vi "Filter for Reports.vi"(7 "Action class name (\"\" = Disable)":string, 8 "error in (no error)":errorcluster, 9 "Type filter (Report = Disable)":T1, 10 "Action Number(<0 = Disable)":i32=-1, 11 "Project Builder in":refnum<class "Project Builder.lvclass">) -> (0 "error out":errorcluster, 1 "Match Found?":bool, 2 "Match Count":i32, 3 "Filtered Reports":T2[](array[typedef]) {"Time End" format="%<%x %.3X>T"; "Time Start" format="%<%x %.3X>T"})   [LabVIEW 2020, in "ProjectBuilder.lvlib" / "Project Builder.lvclass"]
uses:
  Project Builder.lvclass
  Data/Report Data/Report Data.lvclass
  Action/Project Action/Project Action.lvclass
  Ctl/Ctl_Build Steps.ctl
  ProjectBuilder.lvlib
  Ctl/Ctl_Action Result.ctl
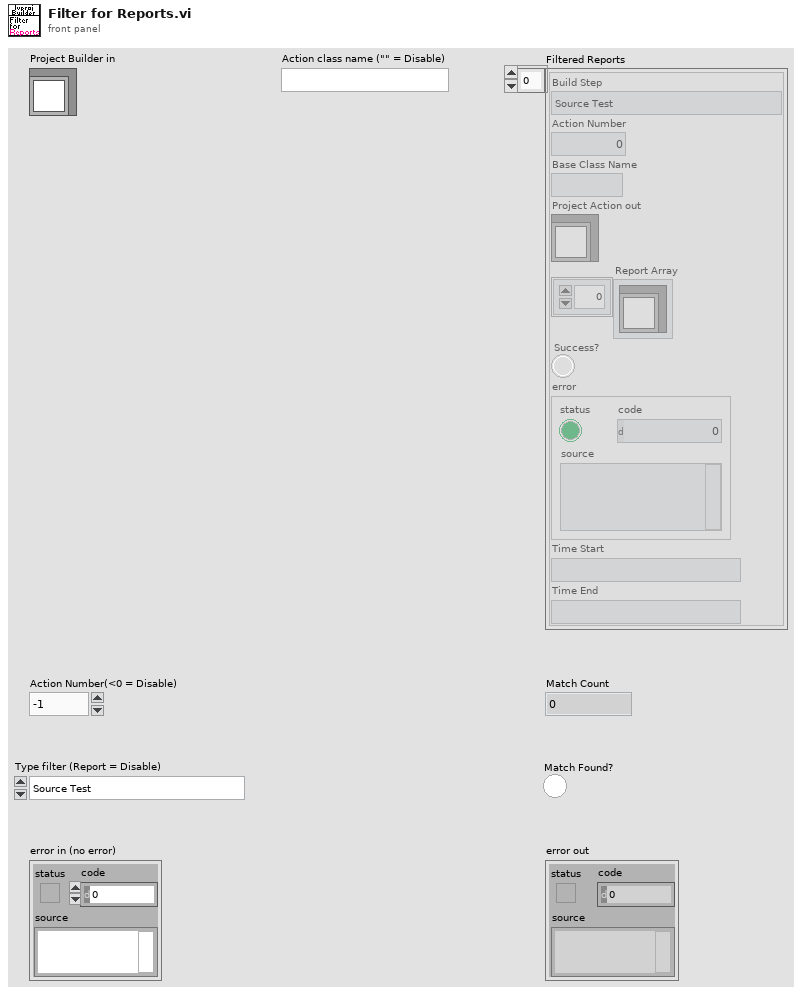
[diagram p1: front panel]
types:
  T1 = typedef "ProjectBuilder.lvlib/Ctl_Build Steps.ctl" = enum16{"Source Test", "Build", "Post-Build Test", "Deploy", "Report"}
  T2 = typedef "ProjectBuilder.lvlib/Ctl_Action Result.ctl" = cluster{"Build Step":T1, "Action Number":i32, "Base Class Name":string, "Project Action out":refnum<class "Project Action.lvclass">, "Report Array":refnum<class "Report Data.lvclass">[], "Success?":bool, "error":errorcluster, "Time Start":timestamp, "Time End":timestamp}
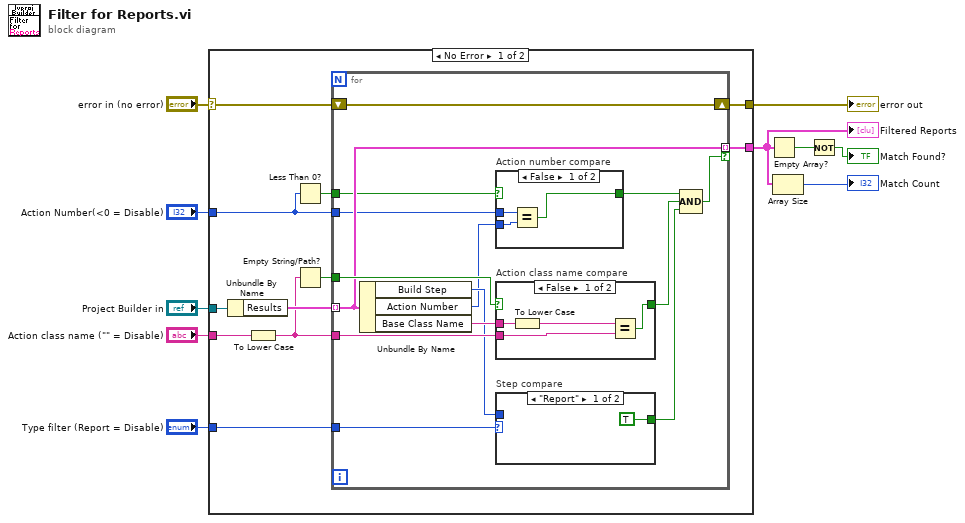
[diagram p0: block diagram]
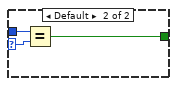
[diagram p3: hidden frame]
diagram:
  n1 = case shown="No Error" "error in (no error)" {
    selector: "error in (no error)" -> [w14 w49]
    tunnel: [w13 w49] -> w9
    tunnel: "Project Builder in" -> [w21 _]
    tunnel: "Action class name (\"\" = Disable)" -> [w19 _]
    tunnel: [w16 _] -> w4
    tunnel: "Type filter (Report = Disable)" -> [w15 _]
    tunnel: "Action Number(<0 = Disable)" -> [w11 _]
    frame No Error {
      n2 = Unbundle By Name(w21) -> ("Results"=w20:T2[])
      n3 = To Lower Case(string=w19) -> (all lower case string=w18:string)
      n4 = Less Than 0?(x=w11) -> (x < 0?=w12:bool)
      n5 = Empty String/Path?(string/path=w18) -> (empty?=w17:bool)
      n6 = for {
        tunnel: w20 -> [w31] mode=indexing
        tunnel: w18 -> [w33]
        tunnel: w17 -> [w34]
        tunnel: [w31] -> w16 mode=indexing if=w30
        tunnel: w15 -> [w29]
        shift-right: [w26] -> w13
        shift-left: w14 -> [w26]
        tunnel: w12 -> [w25]
        tunnel: w11 -> [w23]
        n7 = Unbundle By Name(w31) -> ("Build Step"=w27:T1, "Action Number"=w22:i32, "Base Class Name"=w35:string)
        n8 = case "Action number compare" shown="False" w25 {
          selector: w25 -> [_ w39]
          tunnel: [w36 w39] -> w24
          tunnel: w23 -> [w38 _]
          tunnel: w22 -> [w37 _]
          frame False {
            n9 = Equal?(x=w38, y=w37) -> (x = y?=w36:bool)
          }
          frame True {
          }
        }
        n10 = case "Action class name compare" shown="False" w34 {
          selector: w34 -> [_ w48]
          tunnel: w35 -> [w47 _]
          tunnel: w33 -> [w45 _]
          tunnel: [w44 w48] -> w32
          frame False {
            n11 = To Lower Case(string=w47) -> (all lower case string=w46:string)
            n12 = Equal?(x=w46, y=w45) -> (x = y?=w44:bool)
          }
          frame True {
          }
        }
        n13 = case "Step compare" shown="\"Report\"" w29 {
          selector: w29 -> [_ w43]
          tunnel: [TRUE w42] -> w28
          tunnel: w27 -> [_ w41]
          frame "Report" {
          }
          frame Default {
            n14 = Equal?(x=w41, y=w43) -> (x = y?=w42:bool)
          }
        }
        n15 = Compound Arithmetic op=AND(w24, w32, w28) -> (w30:bool)
      }
    }
    frame Error {
    }
  }
  "error out" <- w9
  "Filtered Reports" <- w4
  n16 = Empty Array?(array=w4) -> (empty?=w6:bool)
  n17 = Array Size(array=w4) -> (size(s)=→"Match Count":i32)
  n18 = Not(x=w6) -> (.not. x?=→"Match Found?":bool)
